vi "Example Graph - Position Callback.vi"(4 "Position":refnum<user-event>, 5 "Event Data":cluster{"sender":refnum<k24>, "position":i16}, 6 "Control Ref":refnum<k24>, 7 "Event Common Data":T1) -> ()   [LabVIEW 2010]
uses:
  C:/tf/play/labview/Tinkerforge.dll
  Tinkerforge.dll
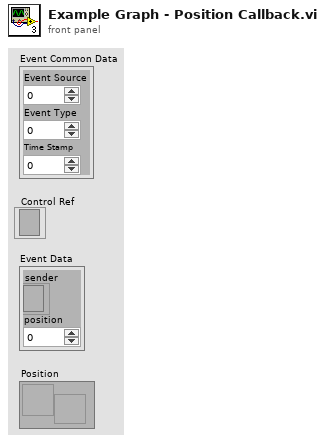
[diagram p1: front panel]
types:
  T1 = cluster{"Event Source":i32, "Event Type":u32, "Time Stamp":u32}
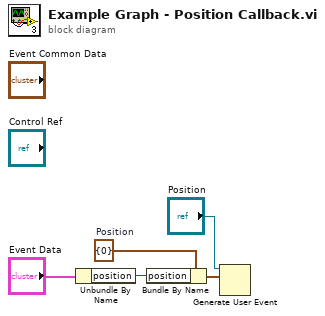
[diagram p0: block diagram]
diagram:
  w2 = cluster{"position":i16} {"position"=0}  # Position
  n1 = Unbundle By Name("Event Data") -> ("position"=w3:i16)
  n2 = Bundle By Name(cluster=w2, "position"=w3) -> (w4:cluster{"position":i16})
  n3 = Generate User Event(user event="Position", event data cluster=w4) -> ()  [unwired: 1 in, 2 out]
